vi "Target.vi"() -> ()   [LabVIEW 2025]
uses:
  <vilib>/Platform/TimedLoop/XDataNode/timing_clust.ctl
  <vilib>/Platform/TimedLoop/XDataNode/nitl_modes.ctl
  <vilib>/Platform/TimedLoop/XDataNode/wakeup.ctl
  <vilib>/rvi/Emulation/niFpgaSctlEmulationGetInTimedLoop.vi
  <vilib>/rvi/Emulation/niFpgaEmulationReportErrorSimple.vi
  <vilib>/rvi/Emulation/niFpgaGetClockAttributes.vi
  <vilib>/rvi/Emulation/niFpgaCriticalErrorInLSC.vi
  <vilib>/rvi/linearAlgebra/MatrixMultiply/simVIs/SubVI/nifxpla_MatrixMultiply_SimMatrixSizes.vi
  <vilib>/rvi/linearAlgebra/MatrixMultiply/simVIs/SubVI/nifxpla_MatrixMultiply_Sim4WireAdapterVector.vi
  <vilib>/rvi/linearAlgebra/MatrixMultiply/simVIs/SubVI/nifxpla_MatrixMultiply_SimFrameHandShake.vi
  <vilib>/rvi/linearAlgebra/MatrixMultiply/simVIs/SubVI/nifxpla_MatrixMultiply_SimEndlessCounter.vi
  <vilib>/rvi/linearAlgebra/MatrixMultiply/simVIs/SubVI/nifxpla_MatrixMultiply_SimVectorDataBuffer.vi
  <vilib>/rvi/ClientSDK/Core/DevComputerLib/Private/Multiply(dfxp64).vi
  <vilib>/rvi/ClientSDK/Core/DevComputerLib/Private/Dfxp128ToDfxp256.vi
  <vilib>/rvi/ClientSDK/Core/DevComputerLib/Private/Add(dfxp256).vi
  <vilib>/rvi/ClientSDK/Core/DevComputerLib/Private/Subtract(dfxp256).vi
  <vilib>/rvi/ClientSDK/Core/DevComputerLib/Private/ToDfxp64(dfxp256).vi
  <vilib>/platform/TimedLoop/XDataNode/XDataNode.xnode
  <vilib>/rvi/linearAlgebra/MatrixMultiply/XNode/nifxpla_MatrixMultiply.xnode
  <vilib>/rvi/linearAlgebra/MatrixMultiply/simVIs/nifxpla_MatrixMultiply_SimTemplateEinEout.vi
  <vilib>/rvi/linearAlgebra/MatrixMultiply/simVIs/nifxpla_MatrixMultiply_SimTemplateEinVout.vi
  <vilib>/rvi/linearAlgebra/MatrixMultiply/simVIs/nifxpla_MatrixMultiply_SimTemplateVinEout.vi
  <vilib>/rvi/linearAlgebra/MatrixMultiply/simVIs/nifxpla_MatrixMultiply_SimTemplateVinVout.vi
  <vilib>/Platform/TimedLoop/XDataNode/XDNodeRunTimeDep.lvlib
panel:
  out "C":fxp<+/-,32,16>[](array[numeric])
  out "Cycle Count":i32
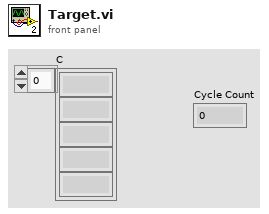
[diagram p1: front panel]
types:
  T1 = typedef "XDNodeRunTimeDep.lvlib/timing_clust.ctl" = cluster{"Expected End [f-1]":u64, "Actual End [f-1]":u64, "Finished Late? [f-1]":bool, "Expected End [i-1]":u64, "Actual End [i-1]":u64, "Finished Late? [i-1]":bool, "Expected Start [i]":u64, "Actual Start [i]":u64, "Expected Start [f]":u64, "Actual Start [f]":u64, "Source Name":string, "Structure Name":string, "Period":i64, "Deadline":i64, "Offset":i64, "Start":i64, "Priority":i32, "Timeout":i32, "Mode":T2, "Wakeup Reason":T3, "Error":errorcluster, "Source Type":string, "Secondary Source Type":string, "Global End Time":u64, "Global Start Time":u64, "Frame Duration":u64, "Iteration Duration":u64, "Assigned CPU":i32, "I/O Scan Engine Mode":u32}
  T2 = typedef "XDNodeRunTimeDep.lvlib/nitl_modes.ctl" = enum32{"No Change", "Process missed periods, maintain original phase", "Discard missed periods, maintain original phase", "Process missed periods, ignore original phase", "Discard missed periods, ignore original phase"}
  T3 = typedef "XDNodeRunTimeDep.lvlib/wakeup.ctl" = enum32{"Normal", "Aborted", "Asynchronous wakeup", "Timing source error", "Timed loop error", "Timeout"}
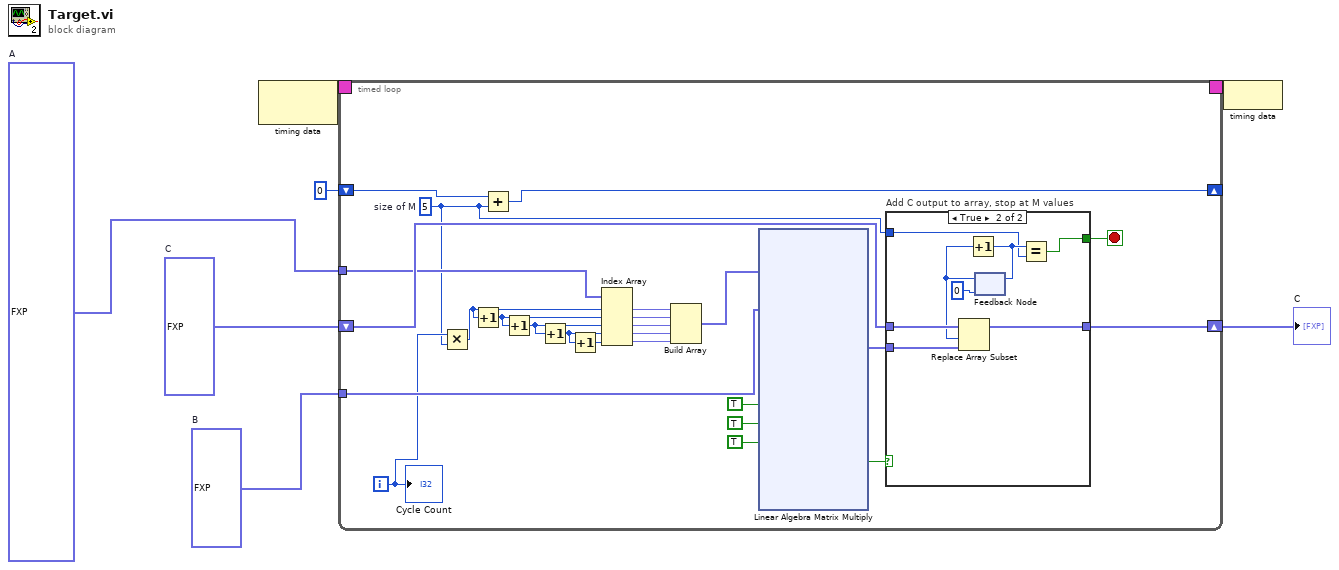
[diagram p0: block diagram]
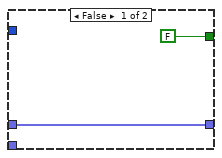
[diagram p2: hidden frame]
diagram:
  w3 = fxp<+/-,32,16>[] [1.0, 2.0, 3.0, 4.0, 5.0, 6.0, 7.0, 8.0, 9.0, 10.0, 11.0, 12.0, 13.0, 14.0, 15.0, 16.0, 17.0, 18.0, 19.0, 20.0, 21.0, 22.0, 23.0, 24.0, 25.0]  # A
  w4 = fxp<+/-,32,16>[] [1.0, 2.0, 3.0, 4.0, 5.0]  # B
  w5 = fxp<+/-,32,16>[] [0.0, 0.0, 0.0, 0.0, 0.0]  # C
  n1 = node-c288() -> (w7:T1)  [unwired: 1 in]
  n2 = timed-loop {
    timing: w7 -> [_]
    timing-out: [_] -> w6
    shift-right: [w31] -> w2
    shift-left: w5 -> [w30]
    tunnel: w4 -> [w27]
    tunnel: w3 -> [w21]
    shift-right: [w23] -> _
    shift-left: 0 ("length") -> [w24]
    i -> [w20]
    stop <- w29 stop-if-true
    w19 = 5  # size of M
    n3 = Multiply(x=w20, y=w19) -> (x*y=w17:i32)
    n4 = Increment(x=w17) -> (x+1=w16:i32)
    n5 = Add(x=w24, y=w19) -> (x+y=w23:i32)
    n6 = Increment(x=w16) -> (x+1=w15:i32)
    n7 = Increment(x=w15) -> (x+1=w14:i32)
    n8 = Increment(x=w14) -> (x+1=w13:i32)
    n9 = Index Array(array=w21, index #1=w17, index #2=w16, index #3=w15, index #4=w14, index #5=w13) -> (element #1=w12:fxp<+/-,32,16>, element #2=w11:fxp<+/-,32,16>, element #3=w10:fxp<+/-,32,16>, element #4=w9:fxp<+/-,32,16>, element #5=w8:fxp<+/-,32,16>)
    n10 = Build Array(w12, w11, w10, w9, w8) -> (w18:fxp<+/-,32,16>[])
    n11 = xnode ("Linear Algebra Matrix Multiply")("ar"=w18, "br"=w27, "a valid"=TRUE, "b valid"=TRUE, "ready for output (T)"=TRUE) -> ("cr"=w26:fxp<+/-,32,16>[], "output valid"=w22:bool)  [unwired: 2 in, 4 out]
    n12 = case "Add C output to array, stop at M values" shown="True" w22 {
      tunnel: w26 -> [_ w38]
      tunnel: [w34 w41] -> w31
      tunnel: w30 -> [w34 w42]
      tunnel: [FALSE w39] -> w29
      tunnel: w19 -> [_ w35]
      frame False {
      }
      frame True {
        n13 = feedback #1(0 ("x")) -> (w37:i32)
        n14 = Replace Array Subset(array=w42, new element=w38, index=w37) -> (w41:fxp<+/-,32,16>[])
        n15 = Increment(x=w37) -> (x+1=w36:i32)
        n16 = feedback-in #1(w36) -> ()
        n17 = Equal?(x=w36, y=w35) -> (x = y?=w39:bool)
      }
    }
    "Cycle Count" <- w20
  }
  "C" <- w2
  n18 = node-c288(w6) -> ()
